vi "Anzahl Span Eingänge dynamisch GD oder Versa Hardware.vi"(6 "Aktion":enum16{"lesen", "schreiben"}(ring), 11 "Anzahl Span in":i32) -> (3 "Anzahl Span out":i32)   [LabVIEW 2020, in "Linearisierung v2.lvlib" / "SpanEinstellungen.lvlib"]
uses:
  SpanEinstellungen.lvlib
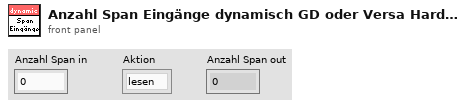
[diagram p1: front panel]
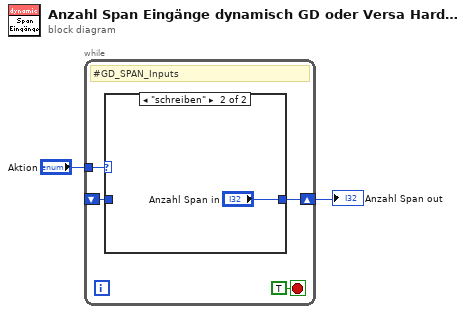
[diagram p0: block diagram]
diagram:
  n1 = while {
    tunnel: "Aktion" -> [w6]
    shift-right: [w4] -> w1
    shift-left: _ -> [w3]
    stop <- TRUE stop-if-true
    # "#GD_SPAN_Inputs"
    n2 = case shown="\"schreiben\"" w6 {
      tunnel: [w7 "Anzahl Span in"] -> w4
      tunnel: w3 -> [w7 _]
      frame "lesen", Default {
      }
      frame "schreiben" {
      }
    }
  }
  "Anzahl Span out" <- w1
